vi "cameraConfNoTrack.vi"(11 "CameraDevRef":T1={"Camera Address"="192.168.0.90", "CameraStatus"={"status"=FALSE, "code"=0, "source"=""}, "Acquire Image Notifier"=refnum}) -> ()   [LabVIEW 2011]
uses:
  <vilib>/Rock Robotics/WPI/Camera/WPI_CameraDevRef.ctl
  <vilib>/Rock Robotics/WPI/Camera/WPI_CameraWhite Balance Values.ctl
  <vilib>/Rock Robotics/WPI/Camera/WPI_CameraExposure Values.ctl
  <vilib>/Rock Robotics/WPI/Camera/WPI_CameraExposure Priority Values.ctl
  <vilib>/Rock Robotics/WPI/Camera/WPI_CameraFrameRate.ctl
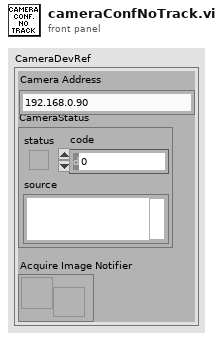
[diagram p1: front panel]
types:
  T1 = typedef "WPI_CameraDevRef.ctl" = cluster{"Camera Address":string, "CameraStatus":errorcluster, "Acquire Image Notifier":refnum<notifier>}
  T2 = typedef "WPI_CameraFrameRate.ctl" = u32
  T3 = typedef "WPI_CameraExposure Priority Values.ctl" = enum16{"None", "Prioritize frame rate", "Prioritize image quality"}
  T4 = typedef "WPI_CameraExposure Values.ctl" = enum16{"Auto", "Flicker-free 50 Hz", "Flicker-free 60 Hz", "Hold current"}
  T5 = typedef "WPI_CameraWhite Balance Values.ctl" = enum16{"Auto", "Fixed indoor", "Fixed outdoor 1", "Fixed outdoor 2", "Fixed fluorescent 1", "Fixed fluorescent 2", "Hold current"}
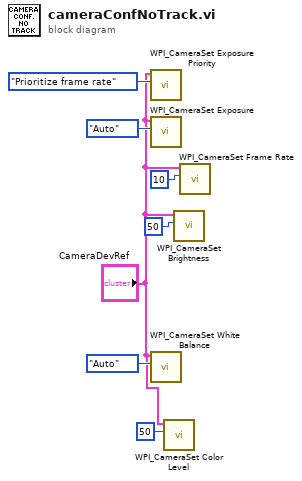
[diagram p0: block diagram]
diagram:
  n1 = call <vilib>:"WPI_CameraSet Exposure Priority.vi"("Exposure Priority"=WPI_CameraExposure_Priority_Values."Prioritize frame rate", "CameraDevRef"="CameraDevRef") -> ()  [unwired: 8 in, 2 out]
  n2 = call <vilib>:"WPI_CameraSet Exposure.vi"("Exposure"=WPI_CameraExposure_Values."Auto", "CameraDevRef"="CameraDevRef") -> ()  [unwired: 8 in, 2 out]
  n3 = call <vilib>:"WPI_CameraSet White Balance.vi"("White Balance"=WPI_CameraWhite_Balance_Values."Auto", "CameraDevRef"="CameraDevRef") -> ()  [unwired: 8 in, 2 out]
  n4 = call <vilib>:"WPI_CameraSet Color Level.vi"("Color Level"=50, "CameraDevRef"="CameraDevRef") -> ()  [unwired: 8 in, 2 out]
  n5 = call <vilib>:"WPI_CameraSet Brightness.vi"("Brightness"=50, "CameraDevRef"="CameraDevRef") -> ()  [unwired: 8 in, 2 out]
  n6 = call <vilib>:"WPI_CameraSet Frame Rate.vi"("Frame Rate (fps)"=T2 10, "CameraDevRef"="CameraDevRef") -> ()  [unwired: 8 in, 2 out]
